vi "ballNearRobot.vi"(8 "Our robots?":bool=TRUE, 10 "Distance":dbl=100.0 format="%#_13g", 11 "IA state":T1={"our_robots"=[], "enemy_robots"=[], "balls"=[], "geometry"={"line_width"=0, "field_length"=0, "field_width"=0, "boundary_width"=0, "referee_width"=0, "goal_width"=0, "goal_depth"=0, "goal_wall_width"=0, "center_circle_radius"=0, "defense_radius"=0, "defense_stretch"=0, "free_kick_from_defense_dist"=0, "penalty_spot_from_field_line_dist"=0, "penalty_line_from_spot_dist"=0}, "IA Judge"={"stage"="", "command"="", "our_goalie_id"=0.0, "enemy_goalie_id"=0.0, "command enum"=enum."Halt", "Time"=enum."Azul"}, "Received Timestamp"=timestamp(0 s since 1904-01-01), "Events"={"Touch"=FALSE, "Ball out"=FALSE, "id touch"=0.0, "Ball out of \nVision"=FALSE, "Ball inside \nGoalie area"=FALSE, "Robot not responding"=FALSE, "Robots responding status"=[1.0, 1.0, 1.0, 1.0, 1.0, 1.0], "Enemy Ball \nPossession"=FALSE, "Pass State"=FALSE, "id end of pass"=0.0, "Kick"=FALSE, "Id ini Possession"=0.0, "Ball Possesion"=FALSE, "Id Possesion"=0.0}}) -> (0 "ID Robot near to ball":u32, 3 "Near to some robot":bool)   [LabVIEW 2017]
uses:
  Intel/Functions Enum.ctl
  Intel/AttackerStates.ctl
  Core/AI Robot.ctl
  Core/AI Ball.ctl
  Core/Field Size.ctl
  Intel/Command Enum.ctl
  Core/AI Judge.ctl
  Util/Events/Events.ctl
  Core/AI Input.ctl
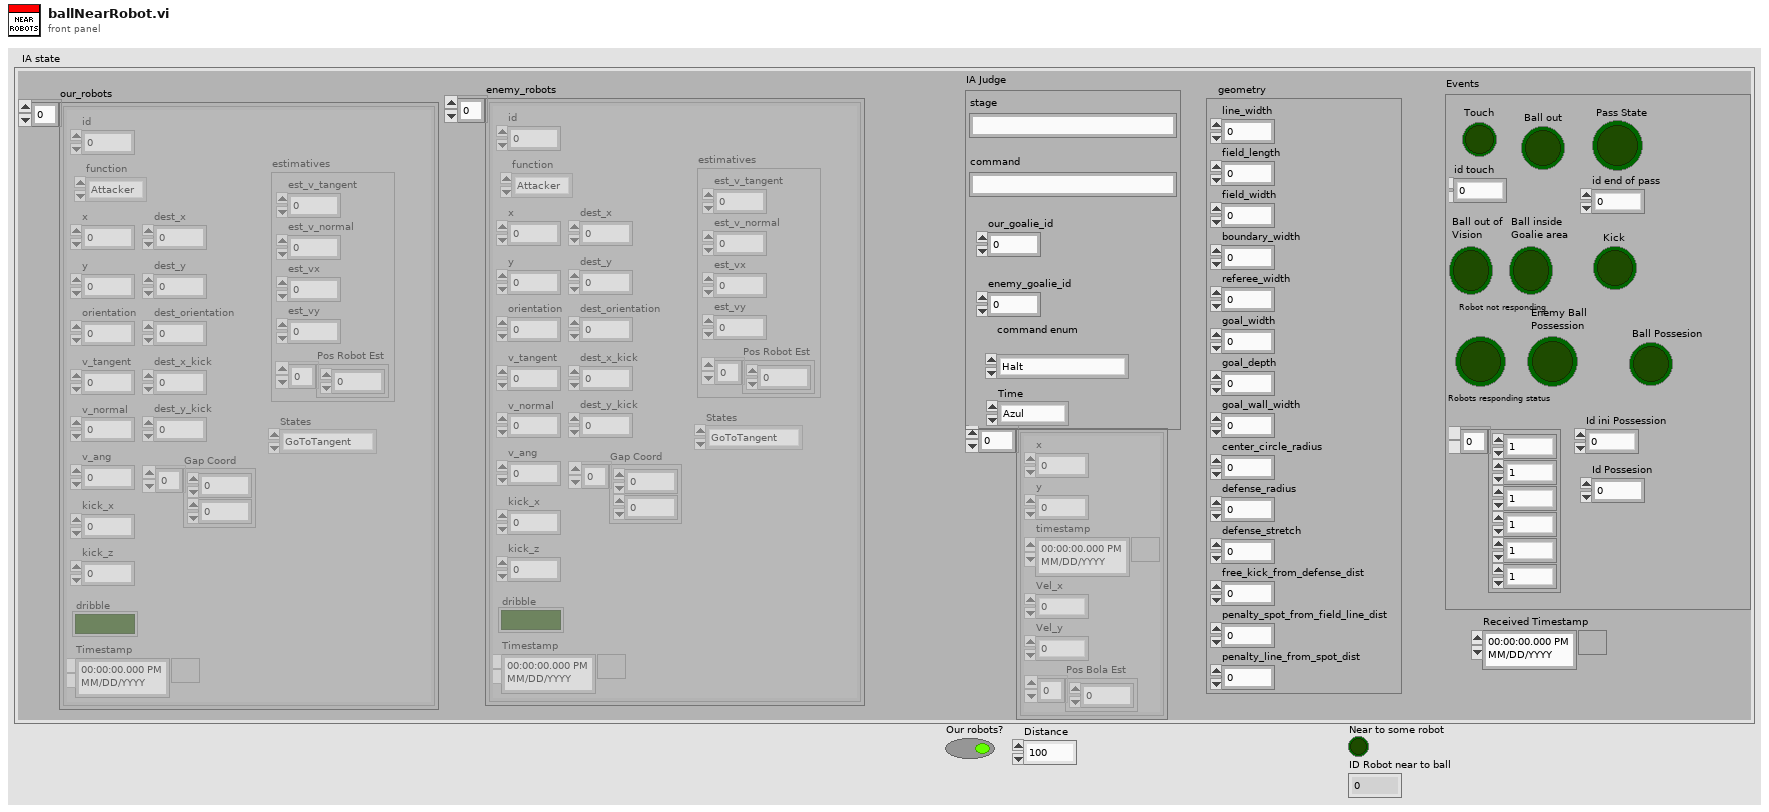
[diagram p1: front panel]
types:
  T1 = typedef "AI Input.ctl" = cluster{"our_robots":T2[], "enemy_robots":T2[], "balls":T5[], "geometry":T6, "IA Judge":T7, "Received Timestamp":timestamp, "Events":T9}
  T2 = typedef "AI Robot.ctl" = cluster{"id":u32, "function":T3, "x":dbl, "y":dbl, "orientation":dbl, "v_tangent":dbl, "v_normal":dbl, "v_ang":dbl, "kick_x":dbl, "kick_z":dbl, "dribble":bool, "Timestamp":timestamp, "dest_x":dbl, "dest_y":dbl, "dest_orientation":dbl, "estimatives":cluster{"est_v_tangent":dbl, "est_v_normal":dbl, "est_vx":dbl, "est_vy":dbl, "Pos Robot Est":dbl[]}, "dest_x_kick":dbl, "dest_y_kick":dbl, "Gap Coord":dbl[], "States":T4}
  T3 = typedef "Functions Enum.ctl" = enum16{"Attacker", "Goalie", "Defender", "Striker", "Goto 0", "Dummy", "Kicker", "ZigZag"}
  T4 = typedef "AttackerStates.ctl" = enum16{"Pass", "GoToTangent", "BallGetting", "GoToKick", ""}
  T5 = typedef "AI Ball.ctl" = cluster{"x":dbl, "y":dbl, "timestamp":timestamp, "Vel_x":dbl, "Vel_y":dbl, "Pos Bola Est":dbl[]}
  T6 = typedef "Field Size.ctl" = cluster{"line_width":u32, "field_length":u32, "field_width":u32, "boundary_width":u32, "referee_width":u32, "goal_width":u32, "goal_depth":u32, "goal_wall_width":u32, "center_circle_radius":u32, "defense_radius":u32, "defense_stretch":u32, "free_kick_from_defense_dist":u32, "penalty_spot_from_field_line_dist":u32, "penalty_line_from_spot_dist":u32}
  T7 = typedef "AI Judge.ctl" = cluster{"stage":string, "command":string, "our_goalie_id":dbl, "enemy_goalie_id":dbl, "command enum":T8, "Time":enum16{"Azul", "Amarelo"}}
  T8 = typedef "Command Enum.ctl" = enum16{"Halt", "Stop", "Force Start", "PKA Normal Start", "Prepare Kickoff Ally", "PKE Normal Start", "Prepare Kickoff Enemy", "Prepare Penalty Ally", "PPA Normal Start", "Prepare Penalty Enemy", "PPE Normal Start", "Direct Free Enemy", "Direct Free Ally", "Indirect Free Enemy", "Indirect Free Ally", "Timeout Enemy", "Timeout Ally", "Goal Enemy", "Goal Ally", "Ball Placement Enemy", "Ball Placement Ally", "Normal Half Time", "Extra Time Break", "Extra Half Time", "None", "Post Game"}
  T9 = typedef "Events.ctl" = cluster{"Touch":bool, "Ball out":bool, "id touch":dbl, "Ball out of \nVision":bool, "Ball inside \nGoalie area":bool, "Robot not responding":bool, "Robots responding status":dbl[], "Enemy Ball \nPossession":bool, "Pass State":bool, "id end of pass":dbl, "Kick":bool, "Id ini Possession":dbl, "Ball Possesion":bool, "Id Possesion":dbl}
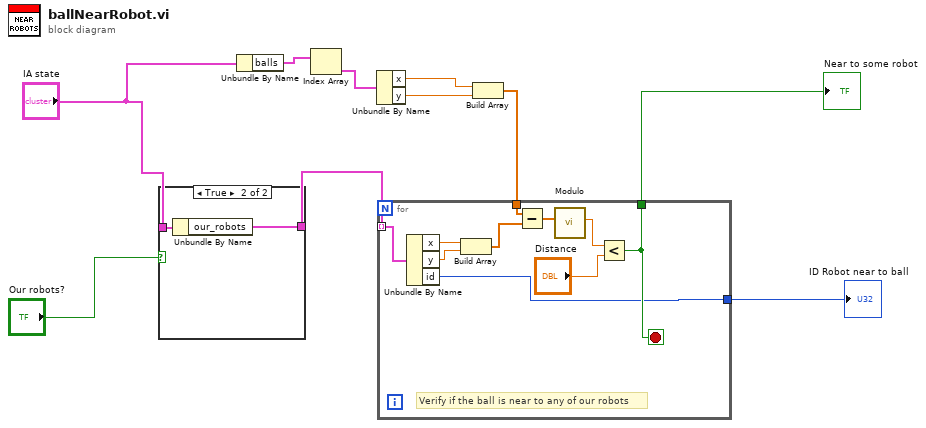
[diagram p0: block diagram]
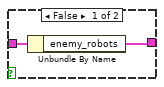
[diagram p2: hidden frame]
diagram:
  n1 = case shown="True" "Our robots?" {
    tunnel: [w11 w14] -> w1
    tunnel: "IA state" -> [w12 w13]
    frame False {
      n2 = Unbundle By Name(w12) -> ("enemy_robots"=w11:T2[])
    }
    frame True {
      n3 = Unbundle By Name(w13) -> ("our_robots"=w14:T2[])
    }
  }
  n4 = Unbundle By Name("IA state") -> ("balls"=w3:T5[])
  n5 = Index Array(array=w3) -> (element=w6:T5)  [unwired: 1 in]
  n6 = Unbundle By Name(w6) -> ("x"=w4:dbl, "y"=w5:dbl)
  n7 = Build Array(w4, w5) -> (w7:dbl[])
  n8 = for {
    tunnel: w1 -> [w24] mode=indexing
    tunnel: w7 -> [w21]
    tunnel: [w16] -> w8
    tunnel: [w15] -> w10
    stop <- w16 stop-if-true
    # "Verify if the ball is near to any of our robots"
    n9 = Unbundle By Name(w24) -> ("x"=w23:dbl, "y"=w22:dbl, "id"=w15:u32)
    n10 = Build Array(w23, w22) -> (w20:dbl[])
    n11 = Subtract(x=w21, y=w20) -> (x-y=w18:dbl[])
    n12 = call "Modulo.vi"("2D vector"=w18) -> ("Modulo"=w17:dbl)  [unwired: 10 in]
    n13 = Less?(x=w17, y="Distance") -> (x < y?=w16:bool)
  }
  "Near to some robot" <- w8
  "ID Robot near to ball" <- w10
